vi "formatObjectInfo.vi"(8 "POI":T2[](array[typedef]), 9 "extent":T2[](array[typedef]), 10 "origin":T2[](array[typedef]), 11 "selectedObj":T1) -> (3 "displayString":string)   [LabVIEW 2015]
uses:
  <vilib>/Utility/miscctls.llb/LV3DPointTypeDef.ctl
  processedObjectInfo.ctl
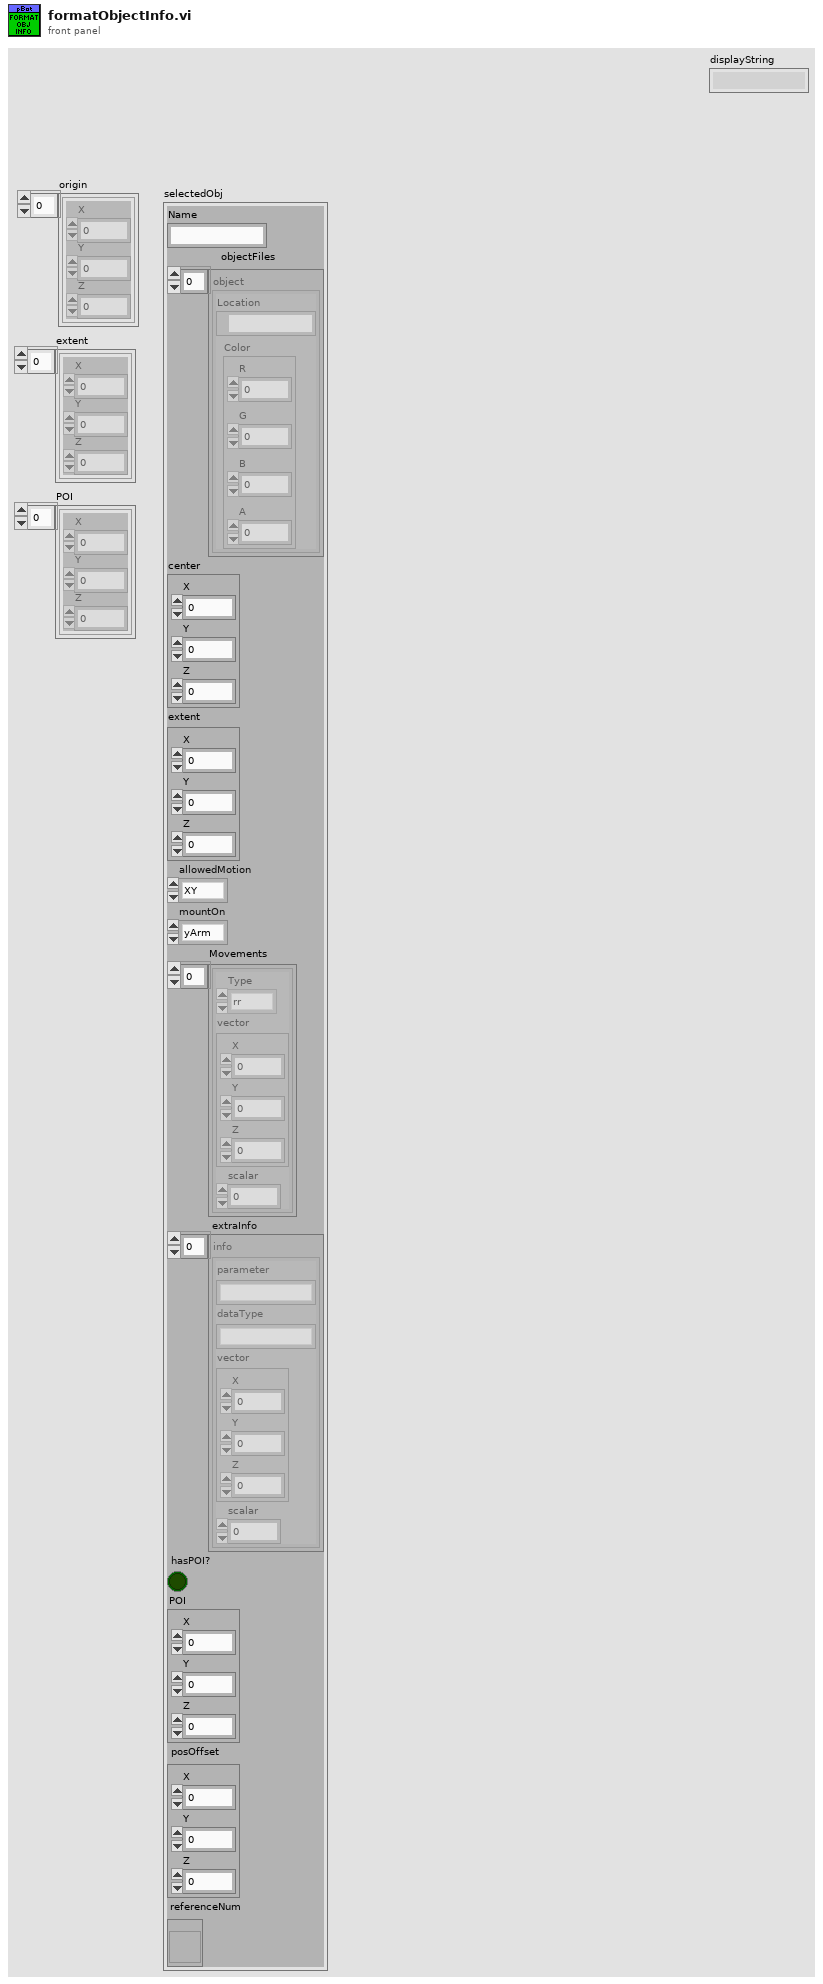
[diagram p1: front panel]
types:
  T1 = typedef "processedObjectInfo.ctl" = cluster{"Name":string, "objectFiles":cluster{"Location":path, "Color":cluster{"R":dbl, "G":dbl, "B":dbl, "A":dbl}}[], "center":cluster{"X":dbl, "Y":dbl, "Z":dbl}, "extent":cluster{"X":dbl, "Y":dbl, "Z":dbl}, "allowedMotion":enum16{"XY", "Z"}, "mountOn":enum16{"yArm", "breadBoard"}, "Movements":cluster{"Type":enum16{"rr", "ra", "tr", "ta"}, "vector":cluster{"X":dbl, "Y":dbl, "Z":dbl}, "scalar":dbl}[], "extraInfo":cluster{"parameter":string, "dataType":string, "vector":cluster{"X":dbl, "Y":dbl, "Z":dbl}, "scalar":dbl}[], "hasPOI?":bool, "POI":cluster{"X":dbl, "Y":dbl, "Z":dbl}, "posOffset":cluster{"X":dbl, "Y":dbl, "Z":dbl}, "referenceNum":refnum<vi>}
  T2 = typedef "LV3DPointTypeDef.ctl" = cluster{"X":sgl, "Y":sgl, "Z":sgl}
  T3 = cluster{"parameter":string, "dataType":string, "vector":cluster{"X":dbl, "Y":dbl, "Z":dbl}, "scalar":dbl}[]
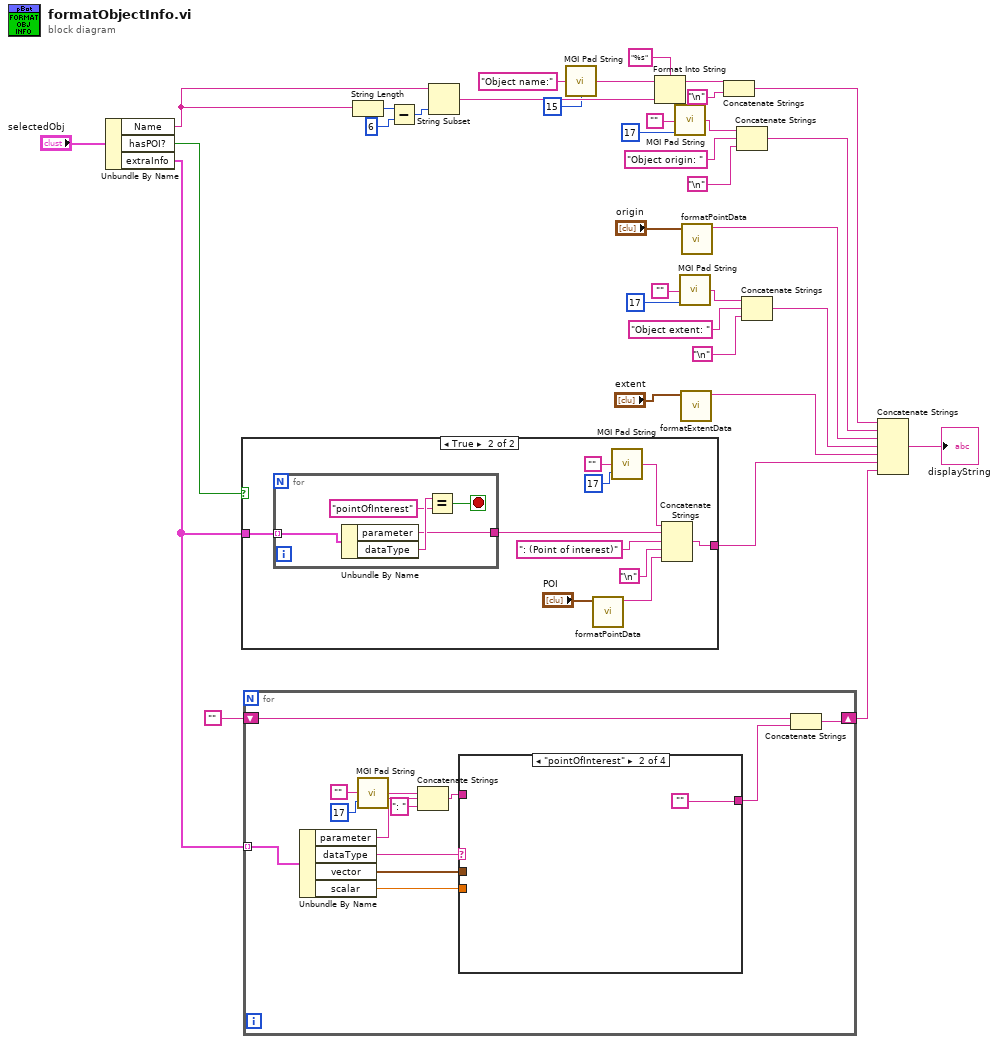
[diagram p0: block diagram]
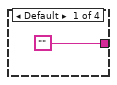
[diagram p2: hidden frame]
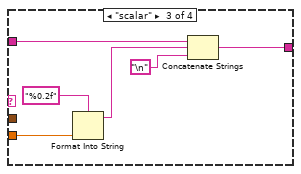
[diagram p3: hidden frame]
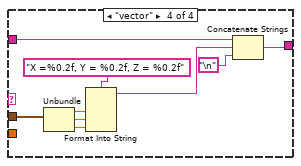
[diagram p4: hidden frame]
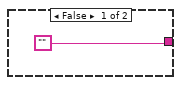
[diagram p5: hidden frame]
diagram:
  n1 = Unbundle By Name("selectedObj") -> ("Name"=w33:string, "hasPOI?"=w5:bool, "extraInfo"=w3:T3)
  n2 = case shown="True" w5 {
    tunnel: w3 -> [_ w42]
    tunnel: ["" w39] -> w4
    frame False {
    }
    frame True {
      n3 = for {
        tunnel: w42 -> [w51] mode=indexing
        tunnel: [w47] -> w38
        stop <- w48 stop-if-true
        n4 = Unbundle By Name(w51) -> ("parameter"=w47:string, "dataType"=w50:string)
        n5 = Equal?(x=w50, y="pointOfInterest" ("initial string")) -> (x = y?=w48:bool)
      }
      n6 = call "formatPointData.vi"("point"="POI") -> ("formatedPointData"=w40:string)  [unwired: 10 in]
      n7 = call <userlib>:"MGI Pad String.vi"("String In"="", "End Length"=u32 17) -> ("String Out"=w45:string)  [unwired: 13 in]
      n8 = Concatenate Strings(w45, w38, ": (Point of interest)" ("initial string"), "\n", w40) -> (w39:string)
    }
  }
  n9 = for {
    tunnel: w3 -> [w64] mode=indexing
    shift-right: [w52] -> w1
    shift-left: "" -> [w53]
    n10 = Unbundle By Name(w64) -> ("parameter"=w59:string, "dataType"=w63:string, "vector"=w55:cluster{"X":dbl, "Y":dbl, "Z":dbl}, "scalar"=w56:dbl)
    n11 = call <userlib>:"MGI Pad String.vi"("String In"="", "End Length"=u32 17) -> ("String Out"=w60:string)  [unwired: 13 in]
    n12 = Concatenate Strings(w60, w59, ": " ("string")) -> (w58:string)
    n13 = case shown="\"pointOfInterest\"" w63 {
      tunnel: w58 -> [_ _ w70 w76]
      tunnel: w56 -> [_ _ w71 _]
      tunnel: ["" "" w67 w73] -> w54
      tunnel: w55 -> [_ _ _ w81]
      frame Default {
      }
      frame "pointOfInterest" {
      }
      frame "scalar" {
        n14 = Format Into String(format string="%0.2f", w71) -> (resulting string=w69:string)  [unwired: 2 in, 1 out]
        n15 = Concatenate Strings(w70, w69, "\n") -> (w67:string)
      }
      frame "vector" {
        n16 = Unbundle(w81) -> ("X"=w79:dbl, "Y"=w78:dbl, "Z"=w77:dbl)
        n17 = Format Into String(format string="X =%0.2f, Y = %0.2f, Z = %0.2f", w79, w78, w77) -> (resulting string=w75:string)  [unwired: 2 in, 1 out]
        n18 = Concatenate Strings(w76, w75, "\n") -> (w73:string)
      }
    }
    n19 = Concatenate Strings(w53, w54) -> (w52:string)
  }
  n20 = String Length(string=w33) -> (length=w32:i32)
  n21 = Subtract(x=w32, y=6) -> (x-y=w30:i32)
  n22 = String Subset(string=w33, length (rest)=w30) -> (substring=w29:string)  [unwired: 1 in]
  n23 = call <userlib>:"MGI Pad String.vi"("String In"="Object name:" ("initial string"), "End Length"=u32 15) -> ("String Out"=w25:string)  [unwired: 13 in]
  n24 = Format Into String(format string="%s", initial string=w25, w29) -> (resulting string=w22:string)  [unwired: 1 in, 1 out]
  n25 = call <userlib>:"MGI Pad String.vi"("String In"="", "End Length"=u32 17) -> ("String Out"=w19:string)  [unwired: 13 in]
  n26 = call <userlib>:"MGI Pad String.vi"("String In"="", "End Length"=u32 17) -> ("String Out"=w11:string)  [unwired: 13 in]
  n27 = call "formatExtentData.vi"("extent"="extent") -> ("formatedExtentData"=w6:string)  [unwired: 10 in]
  n28 = call "formatPointData.vi"("point"="origin") -> ("formatedPointData"=w15:string)  [unwired: 10 in]
  n29 = Concatenate Strings(w22, "\n") -> (w20:string)
  n30 = Concatenate Strings(w19, "Object origin: " ("initial string"), "\n") -> (w16:string)
  n31 = Concatenate Strings(w11, "Object extent: " ("initial string"), "\n") -> (w8:string)
  n32 = Concatenate Strings(w20, w16, w15, w8, w6, w4, w1) -> (→"displayString":string)
